vi "Make permutations.vi"() -> ()   [LabVIEW 2020]
panel:
  out "Array 3":T1(array[cluster])
  out "size(s)":i32
  out "after":i32
  out "before":i32
  out "Array 2":T2(array[cluster])
  out "Array":cluster{"String":string, "String":string}[](array[cluster])
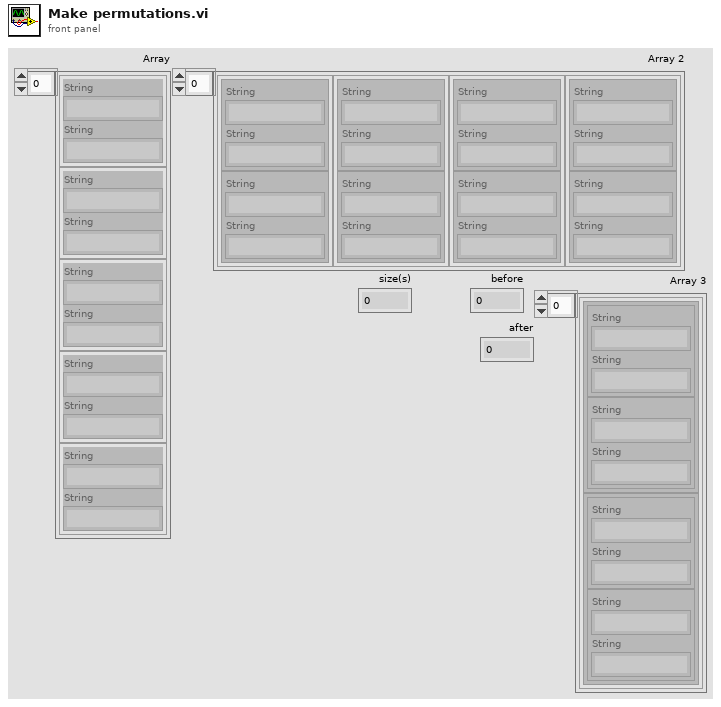
[diagram p1: front panel]
types:
  T1 = cluster{cluster{cluster{"String":string, "String":string}, cluster{"String":string, "String":string}}, cluster{cluster{"String":string, "String":string}, cluster{"String":string, "String":string}}}[]
  T2 = cluster{cluster{"String":string, "String":string}, cluster{"String":string, "String":string}}[]
  T3 = cluster{cluster{"String":string, "String":string}, cluster{"String":string, "String":string}}
  T4 = cluster{cluster{cluster{"String":string, "String":string}, cluster{"String":string, "String":string}}, cluster{cluster{"String":string, "String":string}, cluster{"String":string, "String":string}}}
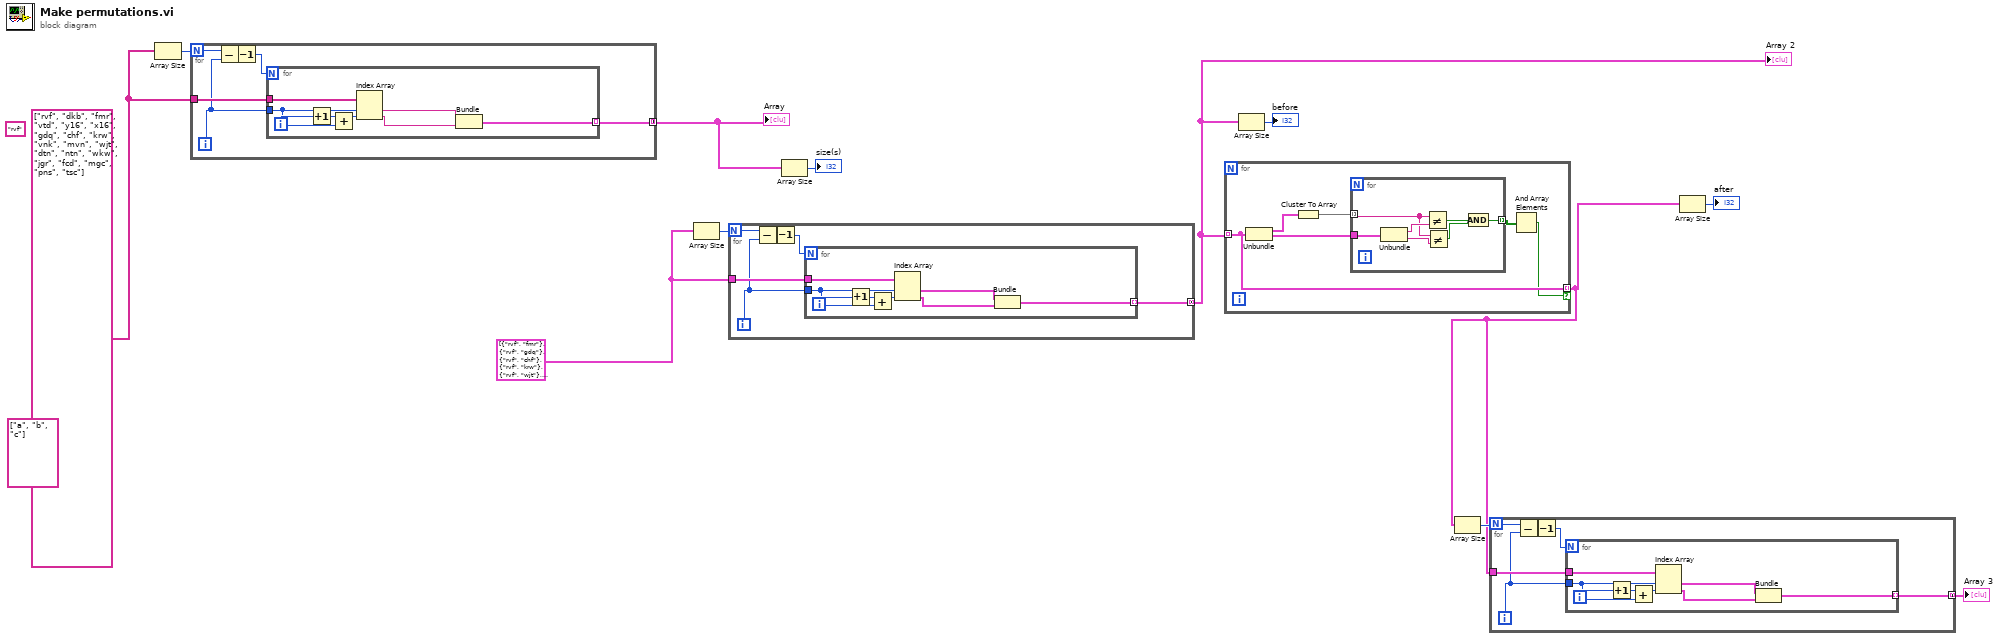
[diagram p0: block diagram]
diagram:
  w5 = cluster{"String":string, "String":string}[] [{"String"="rvf", "String"="fmr"}, {"String"="rvf", "String"="gdq"}, {"String"="rvf", "String"="chf"}, {"String"="rvf", "String"="krw"}, {"String"="rvf", "String"="wjt"}, {"String"="rvf", "String"="dtn"}, {"String"="rvf", "String"="ntn"}, {"String"="rvf", "String"="wkw"}, {"String"="rvf", "String"="fcd"}, {"String"="rvf", "String"="mgc"}, {"String"="rvf", "String"="tsc"}, {"String"="dkb", "String"="vtd"}, {"String"="dkb", "String"="vnk"}, {"String"="dkb", "String"="mvn"}, {"String"="dkb", "String"="ntn"}, {"String"="dkb", "String"="fcd"}, {"String"="dkb", "String"="pns"}, {"String"="fmr", "String"="chf"}, {"String"="fmr", "String"="vnk"}, {"String"="fmr", "String"="mvn"}, {"String"="fmr", "String"="wjt"}, {"String"="fmr", "String"="ntn"}, {"String"="fmr", "String"="fcd"}, {"String"="fmr", "String"="pns"}, {"String"="fmr", "String"="tsc"}, {"String"="vtd", "String"="gdq"}, {"String"="vtd", "String"="chf"}, {"String"="vtd", "String"="vnk"}, {"String"="vtd", "String"="wjt"}, {"String"="vtd", "String"="dtn"}, {"String"="vtd", "String"="ntn"}, {"String"="vtd", "String"="wkw"}, {"String"="vtd", "String"="fcd"}, {"String"="vtd", "String"="mgc"}, {"String"="vtd", "String"="tsc"}, {"String"="y16", "String"="wkw"}, {"String"="y16", "String"="jgr"}, {"String"="x16", "String"="wkw"}, {"String"="x16", "String"="jgr"}, {"String"="gdq", "String"="vnk"}, {"String"="gdq", "String"="mvn"}, {"String"="gdq", "String"="ntn"}, {"String"="gdq", "String"="fcd"}, {"String"="gdq", "String"="pns"}, {"String"="chf", "String"="vnk"}, {"String"="chf", "String"="mvn"}, {"String"="chf", "String"="wjt"}, {"String"="chf", "String"="ntn"}, {"String"="chf", "String"="fcd"}, {"String"="chf", "String"="pns"}, {"String"="krw", "String"="ntn"}, {"String"="krw", "String"="fcd"}, {"String"="vnk", "String"="mvn"}, {"String"="vnk", "String"="wjt"}, {"String"="vnk", "String"="dtn"}, {"String"="vnk", "String"="ntn"}, {"String"="vnk", "String"="wkw"}, {"String"="vnk", "String"="fcd"}, {"String"="vnk", "String"="mgc"}, {"String"="vnk", "String"="tsc"}, {"String"="mvn", "String"="dtn"}, {"String"="mvn", "String"="ntn"}, {"String"="mvn", "String"="wkw"}, {"String"="mvn", "String"="fcd"}, {"String"="mvn", "String"="mgc"}, {"String"="mvn", "String"="tsc"}, {"String"="wjt", "String"="ntn"}, {"String"="wjt", "String"="fcd"}, {"String"="wjt", "String"="pns"}, {"String"="wjt", "String"="tsc"}, {"String"="dtn", "String"="fcd"}, {"String"="dtn", "String"="pns"}, {"String"="ntn", "String"="fcd"}, {"String"="ntn", "String"="pns"}, {"String"="ntn", "String"="tsc"}, {"String"="wkw", "String"="pns"}, {"String"="jgr", "String"="fcd"}, {"String"="jgr", "String"="mgc"}, {"String"="fcd", "String"="pns"}, {"String"="fcd", "String"="tsc"}, {"String"="mgc", "String"="pns"}] ("Array 2")
  (unwired) "rvf" ("String")
  (unwired) string[] ["a", "b", "c"] ("Array 4")
  w10 = string[] ["rvf", "dkb", "fmr", "vtd", "y16", "x16", "gdq", "chf", "krw", "vnk", "mvn", "wjt", "dtn", "ntn", "wkw", "jgr", "fcd", "mgc", "pns", "tsc"] ("Array 4")
  n1 = Array Size(array=w10) -> (size(s)=w12:i32)
  n2 = for {
    N: w12 -> [w17]
    tunnel: w10 -> [w18]
    tunnel: [w13] -> w4 mode=concatenating
    i -> [w15]
    n3 = Subtract(x=w17, y=w15) -> (x-y=w16:i32)
    n4 = Decrement(x=w16) -> (x-1=w14:i32)
    n5 = for {
      N: w14 -> [_]
      tunnel: w18 -> [w26]
      tunnel: w15 -> [w20]
      tunnel: [w19] -> w13 mode=indexing
      i -> [w23]
      n6 = Increment(x=w23) -> (x+1=w22:i32)
      n7 = Add(x=w22, y=w20) -> (x+y=w21:i32)
      n8 = Index Array(array=w26, index #1=w20, index #2=w21) -> (element #1=w25:string, element #2=w24:string)
      n9 = Bundle("String"=w25, "String"=w24) -> (w19:cluster{"String":string, "String":string})  [unwired: 1 in]
    }
  }
  "Array" <- w4
  n10 = Array Size(array=w5) -> (size(s)=w11:i32)
  n11 = for {
    N: w11 -> [w31]
    tunnel: w5 -> [w32]
    tunnel: [w27] -> w9 mode=concatenating
    i -> [w29]
    n12 = Subtract(x=w31, y=w29) -> (x-y=w30:i32)
    n13 = Decrement(x=w30) -> (x-1=w28:i32)
    n14 = for {
      N: w28 -> [_]
      tunnel: w32 -> [w40]
      tunnel: w29 -> [w34]
      tunnel: [w33] -> w27 mode=indexing
      i -> [w37]
      n15 = Increment(x=w37) -> (x+1=w36:i32)
      n16 = Add(x=w36, y=w34) -> (x+y=w35:i32)
      n17 = Index Array(array=w40, index #1=w34, index #2=w35) -> (element #1=w39:cluster{"String":string, "String":string}, element #2=w38:cluster{"String":string, "String":string})
      n18 = Bundle(w39, w38) -> (w33:T3)  [unwired: 1 in]
    }
  }
  "Array 2" <- w9
  n19 = Array Size(array=w4) -> (size(s)=→"size(s)":i32)
  n20 = for {
    tunnel: w9 -> [w42] mode=indexing
    tunnel: [w42] -> w2 mode=indexing if=w41
    n21 = Unbundle(w42) -> (w46:cluster{"String":string, "String":string}, w44:cluster{"String":string, "String":string})
    n22 = Cluster To Array(cluster=w46) -> (array=w45:string[])
    n23 = for {
      tunnel: w45 -> [w50] mode=indexing
      tunnel: w44 -> [w53]
      tunnel: [w47] -> w43 mode=indexing
      n24 = Unbundle(w53) -> ("String"=w52:string, "String"=w51:string)
      n25 = Not Equal?(x=w50, y=w52) -> (x != y?=w48:bool)
      n26 = Not Equal?(x=w50, y=w51) -> (x != y?=w49:bool)
      n27 = And(x=w48, y=w49) -> (x .and. y?=w47:bool)
    }
    n28 = And Array Elements(Boolean array=w43) -> (logical AND=w41:bool)
  }
  n29 = Array Size(array=w9) -> (size(s)=→"before":i32)
  n30 = Array Size(array=w2) -> (size(s)=w3:i32)
  n31 = for {
    N: w3 -> [w58]
    tunnel: w2 -> [w59]
    tunnel: [w54] -> w1 mode=concatenating
    i -> [w56]
    n32 = Subtract(x=w58, y=w56) -> (x-y=w57:i32)
    n33 = Decrement(x=w57) -> (x-1=w55:i32)
    n34 = for {
      N: w55 -> [_]
      tunnel: w59 -> [w67]
      tunnel: w56 -> [w61]
      tunnel: [w60] -> w54 mode=indexing
      i -> [w64]
      n35 = Increment(x=w64) -> (x+1=w63:i32)
      n36 = Add(x=w63, y=w61) -> (x+y=w62:i32)
      n37 = Index Array(array=w67, index #1=w61, index #2=w62) -> (element #1=w66:T3, element #2=w65:T3)
      n38 = Bundle(w66, w65) -> (w60:T4)  [unwired: 1 in]
    }
  }
  "Array 3" <- w1
  n39 = Array Size(array=w2) -> (size(s)=→"after":i32)
